vi "tdo -- V1.vi"() -> ()   [LabVIEW 2021]
uses:
  fft -- data win.ctl
  tdo -- new/Data window.ctl
  agregator -- action.ctl
  interpolation state - real.ctl
  filename-action.ctl
  <vilib>/Analysis/4window.llb/Hanning Window (DBL).vi
  <vilib>/Analysis/4window.llb/Blackman Window (DBL).vi
  <vilib>/Analysis/baseanly.llb/Mean (DBL).vi
  <vilib>/Analysis/8numeric.llb/1D Numeric Integration.vi
  linear interpolation - real -- V2.vi
  <vilib>/Analysis/4window.llb/AllCosWindow (DBL).vi
  <vilib>/Analysis/baseanly.llb/A x B.vi
  <vilib>/Analysis/baseanly.llb/Real A x B.vi
  Q -- check range -- i -- real.vi
  line -- complex.vi
  Q -- check range -- i -- integer.vi
  Q - not nan -- real.vi
  Q - not nan -- integer.vi
  <vilib>/measure/matone.llb/Extract Single Tone Information 1 Chan.vi
  <vilib>/Waveform/WDTOps.llb/WDT Number of Waveform Samples DBL.vi
  <vilib>/Utility/file.llb/Write Delimited Spreadsheet (string).vi
  <vilib>/Analysis/Matrix/Numeric/Conversions/Array To Matrix.vi
  <vilib>/Analysis/Matrix/Numeric/Conversions/Array To Matrix - RA2.vi
  <vilib>/Analysis/baseanly.llb/Inverse Matrix.vi
  <vilib>/Analysis/baseanly.llb/Real Inverse Matrix.vi
  <vilib>/Utility/file.llb/Write Delimited Spreadsheet (DBL).vi
  <vilib>/Analysis/NI_AALPro.lvlib
  <vilib>/measure/NI_MAPro.lvlib
  <vilib>/Analysis/NI_AALBase.lvlib
  <vilib>/Analysis/NI_AAL_SigProc.lvlib
panel:
  in  "ccc":enum32{"Page 1", "Page 2", "Page 3"}(tab)=enum."Page 2"
  out "dt 2":dbl=0.0004 format="%#_6p"
  out "dt 1":dbl=0.0004 format="%#_6p"
  in  "gamma window (sec)":dbl=0.0005 format="%#_6p"
  out "Gamma vs. Field":cluster{dbl[], dbl[]}(graph)
  out "Apmlitude or Pwr. vs. Field":cluster{dbl[], dbl[]}(graph)
  out "Frequency vs. Field":cluster{dbl[], dbl[]}(graph)
  out "Frequency vs. time":waveform(dbl)(graph)={"t0"=timestamp(-0.009969989999999984 s since 1904-01-01), "dt"=2e-05, "Y"=array[5499 elements]}
  out "Progress":dbl(slide)=1.0024540024540025 scale=0.0..1.0
  in  "aaa":enum32{"TDO settings", "file settings"}(tab)
  in  "Power spctr. threshold":dbl=0.0001 format="%.4f"
  in  "Freq. threshold":dbl=30000.0
  in  "window width (s)":dbl=0.0004 format="%#_6p"
  in  "window step (s)":dbl=2e-05 format="%#_6p"
  in  "detection method":T1(ring)
  in  "fit width":i32=9 min=3
  in  "window type":enum16{"Hanning", "Box", "Blackman"}(ring)
  in  "ovewrite file?":bool
  in  "add file suffix":string="_tdo_"
  in  "remove file prefix":string="p_c4_"
  out "first line":string[](array[string])=["012_082225_time 012_082225_field 012_082225_freq 012_082225_amp 012_082225_gamma "]
  in  "Input File":path=path "/Users/arkadyshekhter/Desktop/gdrive/data/Vikram&Shiva&Zoltan--Aug2025/August_2025/082225/p_c4_012_082225.tdms"
  out "Ampl vs. time":waveform(dbl)(graph)={"t0"=timestamp(-0.009969989999999984 s since 1904-01-01), "dt"=2e-05, "Y"=array[5499 elements]}
  in  "bbb":enum32{"data settings", "Field  Settings"}(tab)
  in  "Data window":T2={"Start"=0, "Length"=1000, "Channel numbers"=[0], "Channel names"=["freq", "Field"], "Group name"="p"}
  in  "Bdot Calibration Factor":dbl=3794.0
  out "B dot offset":dbl=1.2807482485038128e-06 format="%.6f"
  in  "Length for Bdot offset, s":dbl=0.009 format="%#_6p"
  in  "Input field format":enum16{"Bdot", "B"}(ring)=enum."B"
  in  "Field correction":dbl=1.0
  in  "Low-pass filter":T3={"Clip IIR filter ramps, in 1/Tc units"=1.0, "Two-pass & flip"=TRUE, "IIR filter specifications"={"Topology"=enum."Off", "Type"=enum."Lowpass", "Order"=1, "Lower Fc"=1e-06, "Upper Fc"=0.0, "PB Ripple"=1.0, "SB Attenuation"=60.0}} {"IIR filter specifications"."PB Ripple" format="%0.2f"; "IIR filter specifications"."Lower Fc" format="%0.2p"; "IIR filter specifications"."SB Attenuation" format="%0.2f"; "IIR filter specifications"."Upper Fc" format="%0.2p"}
  out "Amplitude vs. Field (PWR peak)":cluster{dbl[], "Filtered X":dbl[]}(graph)
  in  "# of threads":i32=4
  out "Field profile":waveform(dbl)(graph)={"t0"=timestamp(-0.009969989999999984 s since 1904-01-01), "dt"=2e-05, "Y"=array[5465 elements]}
  # "Basic NHMFL TDO routine\nv. 0.5       F. F. Balakirev\n\nmessed with by Arkady!"
  # "Background file is either an ASCII *.dat file produced by TDO earlier\nor *.fit file containing single column of polynomial fit coeficients.\n1st row in fit file is a text header, which is ingnored. Result is saved in a \n\"*diff.dat\" file in the output folder\nExample \"PDO1.fit\": \n\nFit y=A_i*x^i, starting with A_0\n3.25637E7\n2132.56863\n-12.60591\n-2.01013\n-0.04452\n-3.23119E-4"
  # "OR"
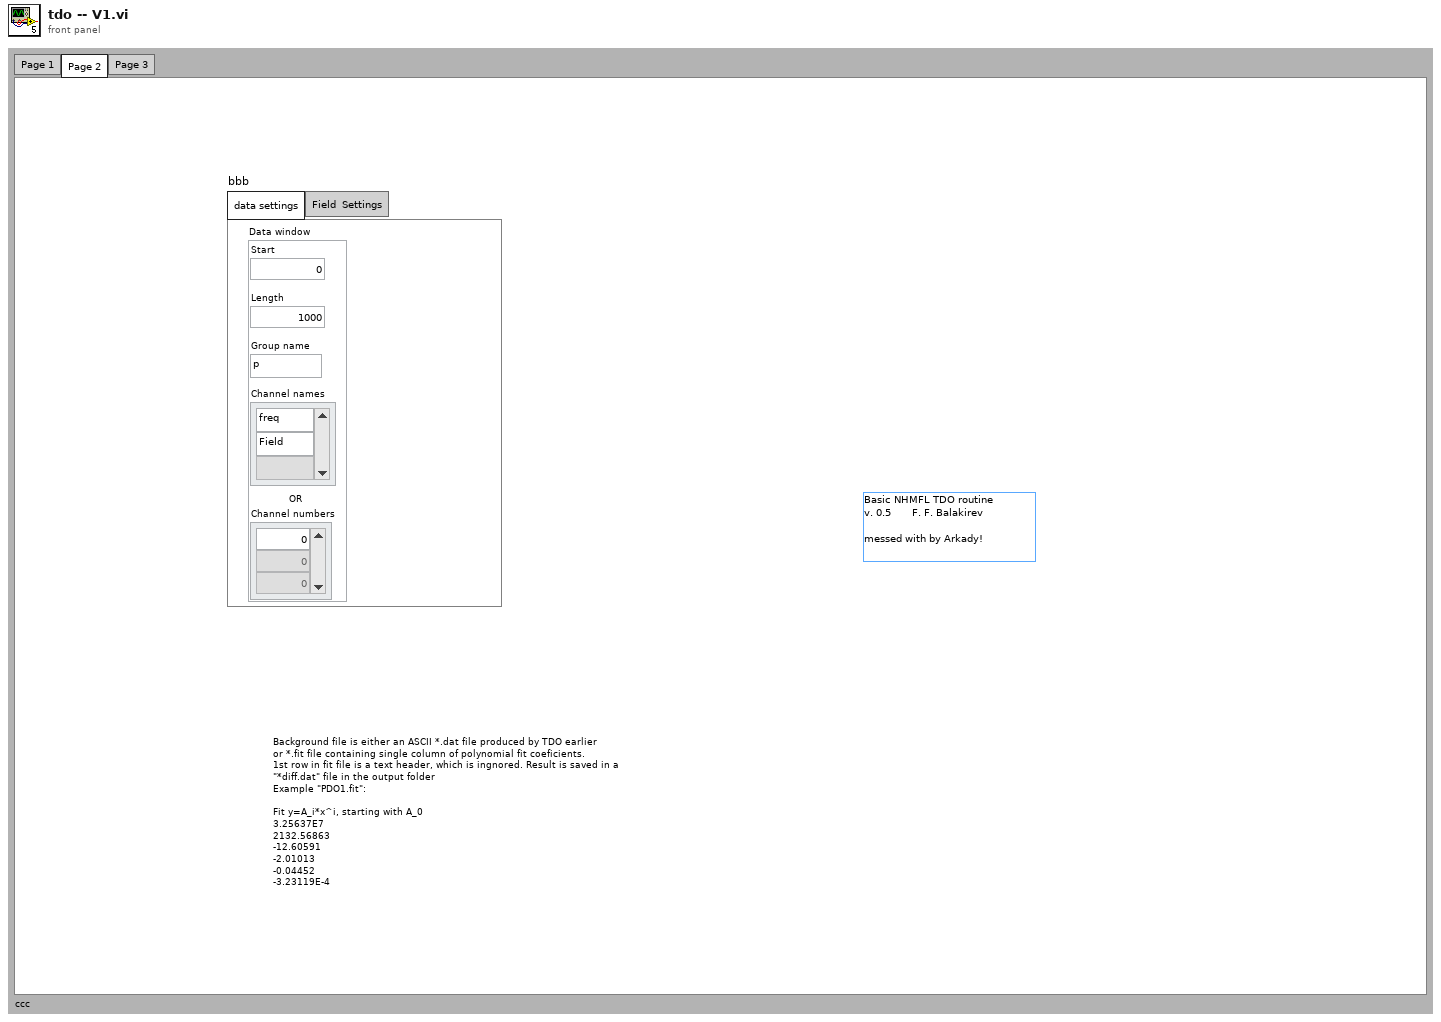
[diagram p1: front panel]
types:
  T1 = enum16{"Power spectrum", "Tone detection", "Peak-to-peak fit"}
  T2 = typedef "fft -- data win.ctl" = cluster{"Start":i64, "Length":i32, "Channel numbers":i64[], "Channel names":string[], "Group name":string}
  T3 = cluster{"Clip IIR filter ramps, in 1/Tc units":dbl, "Two-pass & flip":bool, "IIR filter specifications":cluster{"Topology":enum16{"Off", "Butterworth", "Chebyshev", "Inverse Chebyshev", "Elliptic", "Bessel"}, "Type":enum16{"Lowpass", "Highpass", "Bandpass", "Bandstop"}, "Order":i32, "Lower Fc":dbl, "Upper Fc":dbl, "PB Ripple":dbl, "SB Attenuation":dbl}}
  T4 = typedef "filename-action.ctl" = enum16{"rewrite", "parse", "force pattern", "uniquenum", "get T", "get B", "get ind", "get deg", "get name", "get folder", "get extension", "get basename", "get side", "get setof", "getID", "getIDStock", "remove prefix", "get36thing", "getplain", "getvproj", "getIDStanf"}
  T5 = typedef "interpolation state - real.ctl" = cluster{"Array ":dbl[], "actual size":i32, "requested size":i32}
  T6 = typedef "agregator -- action.ctl" = enum16{"append", "interpolate", "empty!", "force", "init", "scale", "read last"}
  T7 = enum16{"Off", "Butterworth", "Chebyshev", "Inverse Chebyshev", "Elliptic", "Bessel"}
  T8 = typedef "Data window.ctl" = cluster{"Start":i64, "Length":i64, "Channel numbers":i64[], "Channel name":string, "Group name":string}
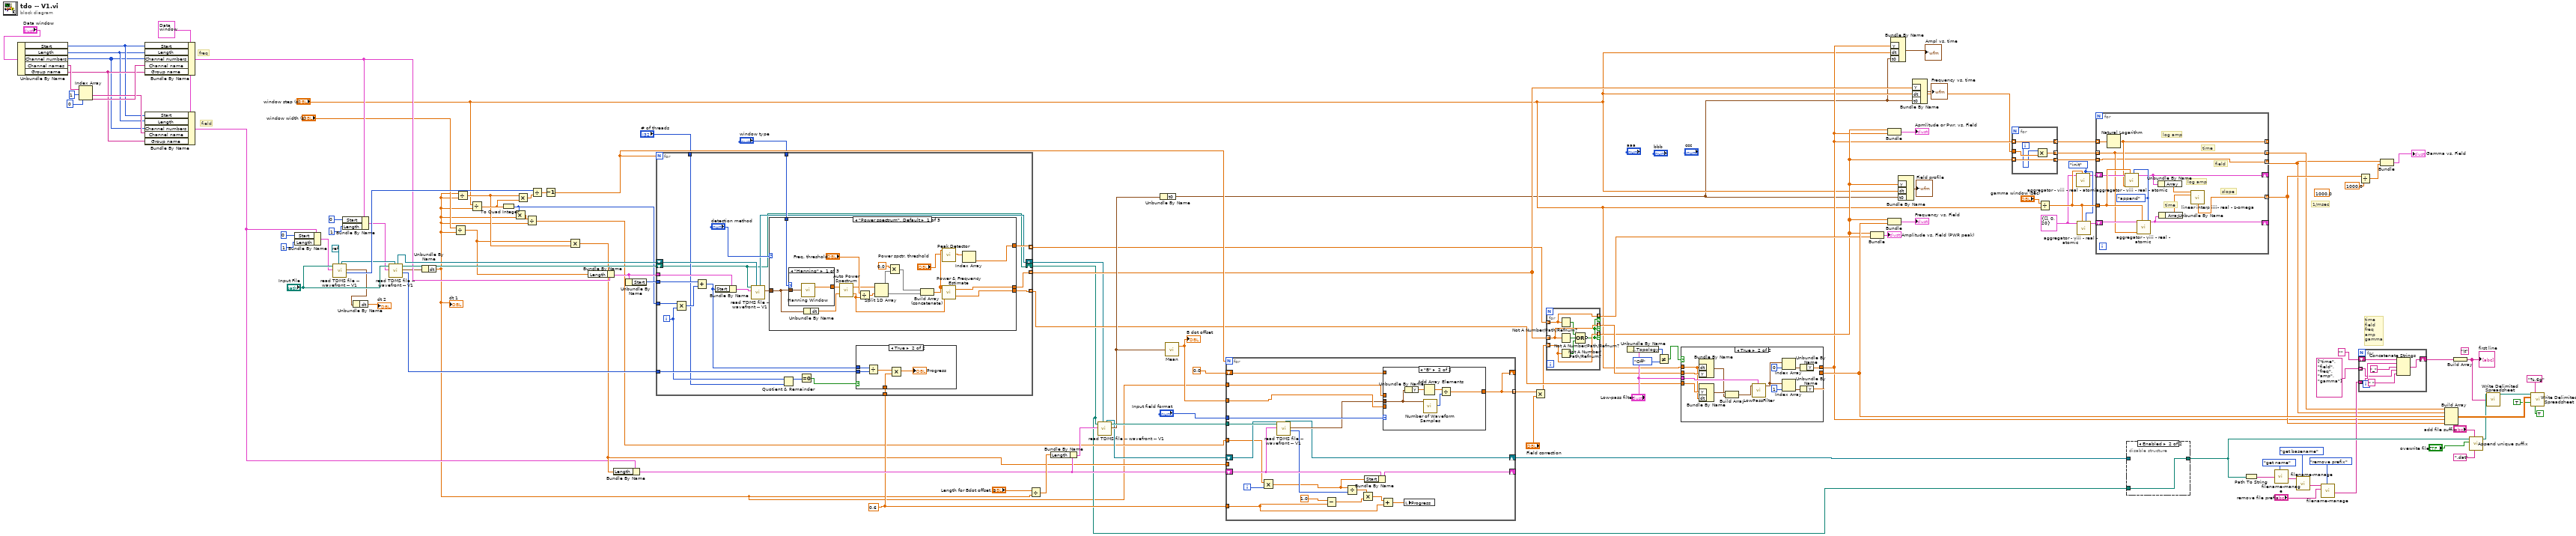
[diagram p0: block diagram]
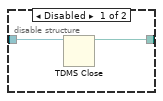
[diagram p2: hidden frame]
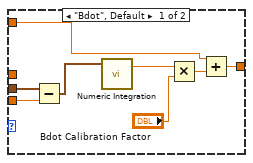
[diagram p3: hidden frame]
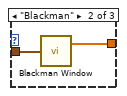
[diagram p6: hidden frame]
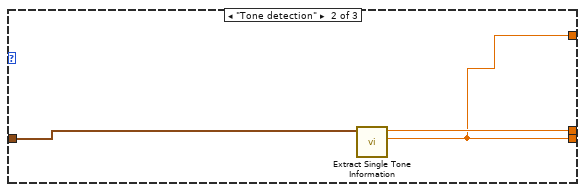
[diagram p8: hidden frame]
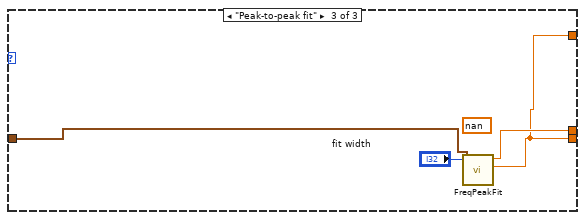
[diagram p9: hidden frame]
diagram:
  (unwired) 1000.0
  (unwired) "\t"
  w44 = T5 {"Array "=[], "actual size"=0, "requested size"=20} ("state IN")
  w48 = agregator_--_action."init" ("aggregator action")
  w77 = 0.6 ("y")
  w9 = T8 {"Start"=0, "Length"=500000, "Channel numbers"=[0], "Channel name"="", "Group name"="Untitled"} ("Data window")
  # "freq"
  # "field"
  # "1/msec"
  # "time \nfield\nfreq\namp\ngamma"
  n1 = Unbundle By Name("Data window") -> ("Start"=w6:i64, "Length"=w5:i32, "Channel numbers"=w4:i64[], "Channel names"=w104:string[], "Group name"=w7:string)
  n2 = Index Array(array=w104, index #1=1 ("index"), index #2=0 ("index")) -> (element #1=w8:string, element #2=w108:string)
  n3 = Bundle By Name(cluster=w9, "Start"=w6, "Length"=w5, "Channel numbers"=w4, "Channel name"=w108, "Group name"=w7) -> (w106:T8)
  n4 = Bundle By Name(cluster=w9, "Start"=w6, "Length"=w5, "Channel numbers"=w4, "Channel name"=w8, "Group name"=w7) -> (w3:T8)
  n5 = Bundle By Name(cluster=w3, "Start"=i64 0, "Length"=i64 1) -> (w101:T8)
  n6 = call "read TDMS file -- wavefront -- V1.vi"("tdms file in"=refnum<k0> refnum, "Data window"=w101, "Input file path"="Input File") -> ("1st channel length"=w115:u64, "Data out"=w103:waveform(dbl), "tdms file out"=w110:refnum<k34>)  [unwired: 5 in, 1 out]
  n7 = Bundle By Name(cluster=w106, "Start"=i64 0, "Length"=i64 1) -> (w100:T8)
  n8 = Unbundle By Name(w103) -> ("dt"=→"dt 2":dbl)
  n9 = call "read TDMS file -- wavefront -- V1.vi"("tdms file in"=w110, "Data window"=w100, "Input file path"="Input File") -> ("1st channel length"=w114:u64, "Data out"=w102:waveform(dbl), "Actual input file path"=w118:path, "tdms file out"=w111:refnum<k34>)  [unwired: 5 in]
  n10 = Unbundle By Name(w102) -> ("dt"=w1:dbl)
  "dt 1" <- w1
  n11 = Divide(x="window width (s)", y=w1) -> (x/y=w67:dbl)
  n12 = Divide(x=w1, y=w1) -> (x/y=w72:dbl)
  n13 = Divide(x="window step (s)", y=w1) -> (x/y=w93:dbl)
  n14 = To Quad Integer(1:w93) -> (0:w66:i64)
  n15 = Multiply(x=w66, y=w1) -> (x*y=w65:dbl)
  n16 = Multiply(x=w72, y=w93) -> (x*y=w83:dbl)
  n17 = Divide(x=w65, y=w1) -> (x/y=w64:dbl)
  n18 = Divide(x=w115, y=w83) -> (x/y=w99:dbl)
  n19 = Decrement(x=w99) -> (x-1=w78:dbl)
  n20 = Multiply(x=w67, y=w72) -> (x*y=w68:dbl)
  n21 = Bundle By Name(cluster=w106, "Length"=w67) -> (w71:T8)
  n22 = Bundle By Name(cluster=w3, "Length"=w68) -> (w84:T8)
  n23 = Unbundle By Name(w71) -> ("Start"=w70:i64)
  n24 = for {
    N: w78 -> [_]
    tunnel: [w138] -> w61 mode=indexing
    tunnel: [w140] -> w62 mode=indexing
    tunnel: [w139] -> w60 mode=indexing
    tunnel: w66 -> [w134]
    tunnel: w114 -> [w137]
    tunnel: w77 -> [w136]
    tunnel: w71 -> [w133]
    tunnel: w70 -> [w132]
    tunnel: "window type" -> [w130]
    tunnel: "# of threads" -> [w123]
    shift-right: [w121] -> w13
    shift-left: w111 -> [w124]
    shift-right: [w120] -> w11
    shift-left: w118 -> [w120]
    i -> [w127]
    n25 = Multiply(x=w134, y=w127) -> (x*y=w128:i64)
    n26 = Add(x=w132, y=w128) -> (x+y=w129:i64)
    n27 = Bundle By Name(cluster=w133, "Start"=w129) -> (w131:T8)
    n28 = call "read TDMS file -- wavefront -- V1.vi"("tdms file in"=w124, "Data window"=w131, "Input file path"=w120) -> ("Data out"=w135:waveform(dbl), "tdms file out"=w121:refnum<k34>)  [unwired: 5 in, 2 out]
    n29 = case shown="\"Power spectrum\", Default" "detection method" {
      tunnel: [w162 w169 w172] -> w140
      tunnel: [w149 w169 w172] -> w139
      tunnel: w135 -> [w161 w170 w175]
      tunnel: [w151 w171 w174] -> w138
      tunnel: w130 -> [w152 _ _]
      frame "Power spectrum", Default {
        n30 = case shown="\"Hanning\"" w152 {
          tunnel: [w165 w167 w168] -> w163
          tunnel: w161 -> [w164 w166 w168]
          frame "Hanning" {
            n31 = call-poly <vilib>:"Hanning Window.vi"("X"=w164) -> ("Windowed X"=w165:dbl[])  [unwired: 1 out]
          }
          frame "Blackman" {
            n32 = call-poly <vilib>:"Blackman Window.vi"("X"=w166) -> ("Windowed X"=w167:dbl[])  [unwired: 1 out]
          }
          frame "Box" {
          }
        }
        n33 = Unbundle By Name(w161) -> ("dt"=w160:dbl)
        n34 = call <vilib>:"Auto Power Spectrum.vi"("dt"=w160, "Signal (V)"=w163) -> ("df"=w150:dbl, "Power Spectrum (V^2 rms)"=w158:dbl[])
        n35 = Divide(x="Freq. threshold", y=w150) -> (x/y=w157:dbl)
        n36 = Split 1D Array(array=w158, index=w157) -> (first subarray=w154:dbl[], second subarray=w156:dbl[])
        n37 = Multiply(x=0.0 ("element"), y=w154) -> (x*y=w153:dbl[])
        n38 = Build Array (concatenate)(w153, w156) -> (w148:dbl[])
        n39 = call <vilib>:"Peak Detector.vi"("threshold"="Power spctr. threshold", "X"=w148) -> ("Amplitudes"=w146:dbl[])  [unwired: 5 in, 4 out]
        n40 = call <vilib>:"Power & Frequency Estimate.vi"("df"=w150, "Power Spectrum (V^2 rms)"=w148) -> ("est power peak"=w162:dbl, "est frequency peak"=w151:dbl)  [unwired: 3 in, 1 out]
        n41 = Index Array(array=w146) -> (element=w149:dbl)  [unwired: 1 in]
      }
      frame "Tone detection" {
        n42 = call-poly <vilib>:"Extract Single Tone Information.vi"("time signal in"=w170) -> ("detected amplitude"=w169:dbl, "detected frequency"=w171:dbl)  [unwired: 3 in, 6 out]
      }
      frame "Peak-to-peak fit" {
        (unwired) nan
        n43 = call "FreqPeakFit.vi"("Peak fit width"="fit width", "Waveform"=w175) -> ("Amplitude"=w172:dbl, "PeakFreqOut"=w174:dbl)  [unwired: 1 in, 5 out]
      }
    }
    n44 = Quotient & Remainder(x=w127, y=w123) -> (x-y*floor(x/y)=w126:i32)  [unwired: 1 out]
    n45 = Equal To 0?(x=w126) -> (x = 0?=w125:bool)
    n46 = case shown="True" w125 {
      tunnel: w137 -> [_ w145]
      tunnel: w136 -> [_ w142]
      tunnel: w129 -> [_ w141]
      frame False {
      }
      frame True {
        n47 = Divide(x=w141, y=w145) -> (x/y=w144:dbl)
        n48 = Multiply(x=w144, y=w142) -> (x*y=→"Progress":dbl)
      }
    }
  }
  n49 = Divide(x="Length for Bdot offset, s", y=w1) -> (x/y=w85:dbl)
  n50 = Bundle By Name(cluster=w84, "Length"=w85) -> (w76:T8)
  n51 = call "read TDMS file -- wavefront -- V1.vi"("tdms file in"=w13, "Data window"=w76, "Input file path"=w11) -> ("Data out"=w75:waveform(dbl), "Actual input file path"=w79:path, "tdms file out"=w74:refnum<k34>)  [unwired: 5 in, 1 out]
  n52 = Unbundle By Name(w75) -> ("t0"=w19:timestamp)
  n53 = call-poly <vilib>:"Mean.vi"("X"=w75) -> ("mean"=w81:dbl)  [unwired: 1 out]
  "B dot offset" <- w81
  n54 = for {
    N: w78 -> [_]
    shift-right: [w196] -> _
    shift-left: w84 -> [w195]
    tunnel: w64 -> [w178]
    tunnel: "Input field format" -> [w194]
    tunnel: w81 -> [w193]
    shift-right: [w192] -> _
    shift-left: 0.0 -> [w191]
    tunnel: [w192] -> w56 mode=indexing
    tunnel: w1 -> [w190]
    tunnel: w79 -> [w189]
    tunnel: w77 -> [w176]
    shift-right: [w180] -> w73
    shift-left: w74 -> [w181]
    tunnel: w68 -> [_]
    i -> [w179]
    n55 = Multiply(x=w178, y=w179) -> (x*y=w177:dbl)
    n56 = call "read TDMS file -- wavefront -- V1.vi"("tdms file in"=w181, "Data window"=w195, "Input file path"=w189) -> ("1st channel length"=w187:u64, "Data out"=w182:waveform(dbl), "tdms file out"=w180:refnum<k34>)  [unwired: 5 in, 1 out]
    n57 = Subtract(x=1.0, y=w176) -> (x-y=w185:dbl)
    n58 = Divide(x=w177, y=w187) -> (x/y=w188:dbl)
    n59 = Multiply(x=w188, y=w185) -> (x*y=w183:dbl)
    n60 = Bundle By Name(cluster=w195, "Start"=w177) -> (w196:T8)
    n61 = Add(x=w183, y=w176) -> (x+y=w184:dbl)
    n62 = case shown="\"B\"" w194 {
      tunnel: w191 -> [w204 _]
      tunnel: [w202 w206] -> w192
      tunnel: w193 -> [w200 _]
      tunnel: w190 -> [_ _]
      tunnel: w182 -> [w198 w205]
      frame "Bdot", Default {
        n63 = Subtract(x=w198, y=w200) -> (x-y=w201:waveform(dbl))
        n64 = call-poly <vilib>:"Numeric Integration.vi"("Input Array"=w201) -> ("result"=w199:dbl)  [unwired: 2 in, 1 out]
        n65 = Multiply(x=w199, y="Bdot Calibration Factor") -> (x*y=w203:dbl)
        n66 = Add(x=w204, y=w203) -> (x+y=w202:dbl)
      }
      frame "B" {
        n67 = Unbundle By Name(w205) -> ("Y"=w209:dbl[])
        n68 = Add Array Elements(numeric array=w209) -> (sum=w207:dbl)
        n69 = call-poly <vilib>:"Number of Waveform Samples.vi"("waveform in"=w205) -> ("number of samples"=w208:i32)  [unwired: 1 in, 9 out]
        n70 = Divide(x=w207, y=w208) -> (x/y=w206:dbl)
      }
    }
    n71 = local write "Progress"(w184) -> ()
  }
  n72 = Multiply(x=w56, y="Field correction") -> (x*y=w54:dbl[])
  n73 = for {
    tunnel: w61 -> [w215] mode=indexing
    tunnel: w54 -> [w214] mode=indexing
    tunnel: w60 -> [w216] mode=indexing
    tunnel: [w216] -> w57 mode=indexing if=w210
    tunnel: [w215] -> w58 mode=indexing if=w210
    tunnel: [w214] -> w52 mode=indexing if=w210
    n74 = Not A Number/Path/Refnum?(number/path/refnum=w216) -> (NaN/Path/Refnum?=w213:bool)
    n75 = Not A Number/Path/Refnum?(number/path/refnum=w215) -> (NaN/Path/Refnum?=w212:bool)
    n76 = Not A Number/Path/Refnum?(number/path/refnum=w214) -> (NaN/Path/Refnum?=w211:bool)
    n77 = Compound Arithmetic op=OR(w213, w212, w211) -> (invert w210:bool)
  }
  n78 = Unbundle By Name("Low-pass filter") -> ("IIR filter specifications.Topology"=w91:T7)
  n79 = Not Equal?(x=w91, y=T7."Off" ("IIR filter specifications.Topology")) -> (x != y?=w90:bool)
  n80 = case shown="True" w90 {
    tunnel: "Low-pass filter" -> [_ w232]
    tunnel: w62 -> [w218 w230]
    tunnel: w58 -> [w217 w231]
    tunnel: "window step (s)" -> [_ w219]
    tunnel: [w217 w221] -> w59
    tunnel: [w218 w220] -> w21
    frame False {
    }
    frame True {
      n81 = Bundle By Name("dt"=w219, "Y"=w231) -> (w228:waveform(dbl))  [unwired: 1 out]
      n82 = Bundle By Name("Y"=w230, "dt"=w219) -> (w229:waveform(dbl))  [unwired: 1 out]
      n83 = Build Array(w229, w228) -> (w227:waveform(dbl)[])
      n84 = call "LowPassFilter.vi"("Low-pass filter"=w232, "signal(s) in"=w227) -> ("signal(s) out"=w226:waveform(dbl)[])  [unwired: 3 in, 6 out]
      n85 = Index Array(array=w226, index=0) -> (element=w223:waveform(dbl))
      n86 = Index Array(array=w226, index=1) -> (element=w222:waveform(dbl))
      n87 = Unbundle By Name(w223) -> ("Y"=w220:dbl[])
      n88 = Unbundle By Name(w222) -> ("Y"=w221:dbl[])
    }
  }
  n89 = Bundle(w52, w57) -> (→"Amplitude vs. Field (PWR peak)":cluster{dbl[], dbl[]})  [unwired: 1 out]
  n90 = Bundle(w52, "Y"=w21) -> (→"Apmlitude or Pwr. vs. Field":cluster{dbl[], "Y":dbl[]})  [unwired: 1 out]
  n91 = Bundle(w52, "Y"=w59) -> (→"Frequency vs. Field":cluster{dbl[], "Y":dbl[]})  [unwired: 1 out]
  n92 = Bundle By Name("Y"=w21, "dt"="window step (s)", "t0"=w19) -> (→"Ampl vs. time":waveform(dbl))  [unwired: 1 out]
  n93 = Bundle By Name("Y"=w52, "dt"="window step (s)", "t0"=w19) -> (→"Field profile":waveform(dbl))  [unwired: 1 out]
  n94 = Bundle By Name("Y"=w61, "dt"="window step (s)", "t0"=w19) -> (→"Frequency vs. time":waveform(dbl))  [unwired: 1 out]
  n95 = for {
    tunnel: w21 -> [w235] mode=indexing
    tunnel: "window step (s)" -> [w237]
    tunnel: [w236] -> w43 mode=indexing
    tunnel: [w235] -> w50 mode=indexing
    tunnel: [w234] -> w46 mode=indexing
    tunnel: w52 -> [w234] mode=indexing
    i -> [w233]
    n96 = Multiply(x=w233, y=w237) -> (x*y=w236:dbl)
  }
  n97 = Divide(x="gamma window (sec)", y="window step (s)") -> (x/y=w49:dbl)
  n98 = call "aggregator - viii - real - atomic.vi"("aggregator action"=w48, "requested size"=w49, "state IN"=w44) -> ("state OUT"=w47:T5)  [unwired: 5 in, 3 out]
  n99 = call "aggregator - viii - real - atomic.vi"("aggregator action"=w48, "requested size"=w49, "state IN"=w44) -> ("state OUT"=w51:T5)  [unwired: 5 in, 3 out]
  n100 = for {
    shift-right: [w244] -> _
    shift-left: w51 -> [w250]
    tunnel: w49 -> [w247]
    tunnel: w50 -> [w249] mode=indexing
    tunnel: w43 -> [w239] mode=indexing
    shift-right: [w245] -> _
    shift-left: w47 -> [w246]
    tunnel: [w241] -> w23 mode=indexing
    tunnel: [w240] -> _ mode=indexing
    tunnel: [w239] -> w15 mode=indexing
    tunnel: w46 -> [w238] mode=indexing
    tunnel: [w238] -> w14 mode=indexing
    w248 = agregator_--_action."append" ("aggregator action")
    # "field"
    # "slope"
    # "time"
    # "log amp"
    # "log amp"
    # "time"
    n101 = Natural Logarithm(1:w249) -> (0:w240:dbl)
    n102 = call "aggregator - viii - real - atomic.vi"("aggregator action"=w248, "requested size"=w247, "number"=w240, "state IN"=w246) -> ("state OUT"=w245:T5)  [unwired: 4 in, 3 out]
    n103 = call "aggregator - viii - real - atomic.vi"("aggregator action"=w248, "requested size"=w247, "number"=w239, "state IN"=w250) -> ("state OUT"=w244:T5)  [unwired: 4 in, 3 out]
    n104 = Unbundle By Name(w245) -> ("Array"=w242:dbl[])
    n105 = Unbundle By Name(w244) -> ("Array"=w243:dbl[])
    n106 = call "linear interp iiii- real - z-omega.vi"("z"=w242, "omega"=w243) -> ("slope"=w241:dbl)  [unwired: 4 in, 9 out]
  }
  n107 = disable-structure shown="Enabled" {
    disable-tunnel: w73 -> [w252 _]
    disable-tunnel: [w251 w253] -> w34
    disable-tunnel: w11 -> [_ w253]
    frame Disabled {
      n108 = TDMS Close(11:w252) -> (3:w251:path)  [unwired: 1 in, 1 out]
    }
    frame Enabled {
    }
  }
  n109 = Path To String(path=w34) -> (string=w32:string)
  n110 = call "filename-manage.vi"("filename-action"=filename-action."get name", "file name IN"=w32) -> ("string OUT"=w31:string)  [unwired: 7 in, 2 out]
  n111 = call "filename-manage.vi"("filename-action"=filename-action."get basename", "file name IN"=w31) -> ("string OUT"=w29:string)  [unwired: 7 in, 2 out]
  n112 = call "filename-manage.vi"("filename-action"=filename-action."remove prefix", "string IN"="remove file prefix", "file name IN"=w29) -> ("string OUT"=w26:string)  [unwired: 6 in, 2 out]
  n113 = Divide(x=w23, y=1000.0) -> (x/y=w22:dbl[])
  n114 = for {
    tunnel: string[] ["time", "field", "freq", "amp", "gamma"] -> [w255] mode=indexing
    shift-right: [w258] -> w24
    shift-left: "" ("format (%.3f)") -> [w259]
    tunnel: w26 -> [w257]
    n115 = Concatenate Strings(w259, w257, "_", w255, " ") -> (w258:string)
  }
  n116 = Bundle(w14, w22) -> (→"Gamma vs. Field":cluster{dbl[], dbl[]})  [unwired: 1 out]
  n117 = Build Array(w15, w14, w59, w21, w23) -> (w97:dbl[][])
  n118 = Build Array(w24) -> (w36:string[])
  "first line" <- w36
  n119 = call "Append unique suffix.vi"("Extention"=".dat", "Suffix"="add file suffix", "ovewrite ?"="ovewrite file?", "Path"=w34) -> ("Path out"=w37:path)  [unwired: 6 in, 1 out]
  n120 = call-poly <vilib>:"Write Delimited Spreadsheet.vi"("file path (dialog if empty)"=w37, "1D data"=w36) -> ("new file path (Not A Path if cancelled)"=w35:path)  [unwired: 12 in, 1 out]
  n121 = call-poly <vilib>:"Write Delimited Spreadsheet.vi"("file path (dialog if empty)"=w35, "format (%.3f)"="%.6g", "2D data"=w97, "append to file? (new file:F)"=TRUE, "transpose? (no:F)"=TRUE) -> ()  [unwired: 9 in, 2 out]
